vi "CanControlOpen.vi"(3 "error in":errorcluster {"code" format="%.0x"}, 4 "CAN Number":u32 max=31 step=1, 5 "Device Handle":u32 format="%x") -> (0 "error out":errorcluster {"code" format="%.0x"}, 2 "CAN Control Handle":u32 format="%x")   [LabVIEW 2011]
doc: "Opens a CAN controller on the specified VCI device."
uses:
  vcilva.dll
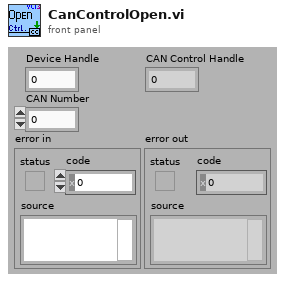
[diagram p1: front panel]
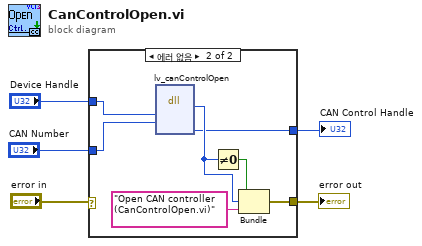
[diagram p0: block diagram]
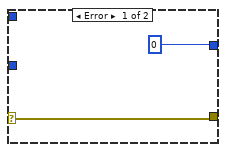
[diagram p2: hidden frame]
diagram:
  n1 = case shown="에러 없음" "error in" {
    selector: "error in" -> [w7 _]
    tunnel: [w7 w14] -> w4
    tunnel: "CAN Number" -> [_ w10]
    tunnel: "Device Handle" -> [_ w9]
    tunnel: [u32 0 ("hCanCtrl") w8] -> w1
    frame Error {
    }
    frame No Error {
      n2 = dll-call lib="vcilva.dll" fn="lv_canControlOpen"("hDevice"=w9, "CanNo"=w10) -> (w11:i32, "hCanCtl"=w8:u32)  [unwired: 6 in, 2 out]
      n3 = Not Equal To 0?(x=w11) -> (x != 0?=w13:bool)
      n4 = Bundle(w13, w11, "Open CAN controller  (CanControlOpen.vi)") -> (w14:errorcluster)  [unwired: 1 in]
    }
  }
  "error out" <- w4
  "CAN Control Handle" <- w1
